vi "GetObjectExternalInterfaces.vi"(8 "Error In":errorcluster, 9 "Label":string, 10 "ThisObject":string, 11 "reference in":refnum<class "AppConfigJSON.lvclass">) -> (0 "Error Out":errorcluster, 1 "ObjectData":T1, 2 "Valid?":bool, 3 "reference out":refnum<class "AppConfigJSON.lvclass">)   [LabVIEW 2021, in "AppConfigJSON.lvclass"]
uses:
  AppConfigJSON.lvclass
  Interface_TAF_IApplicationConfiguration/IApplicationConfiguration/ObjectData.ctl
  d9591dce-848e-416d-bce7-ad181968b3a1.vi
  <vilib>/TriekselSoft/TracerLibrary/TracerLibrary/Tracer/protected/SendMessage.vi
  <vilib>/TriekselSoft/TracerLibrary/TracerLibrary/Tracer/protected/Timestamp.vi
  d9591dce-848e-416d-bce7-ad181968b3a1.vi/f75db090-0877-4668-94fb-75c2140b1617.vi
  <vilib>/TriekselSoft/TracerLibrary/TracerLibrary/Tracer/Tracer_Level-Warning.vi
  <vilib>/JDP Science/JSONtext/Variant to JSON Text.vi
  <vilib>/TriekselSoft/TracerLibrary/TracerLibrary/Tracer/protected/Tracer_ClassAttributes.vi
  <vilib>/JDP Science/JSONtext/LVClass Serializer/JSONtext LVClass Serializer.lvclass
  Interface_TAF_IApplicationConfiguration/IApplicationConfiguration/IApplicationConfiguration.lvclass
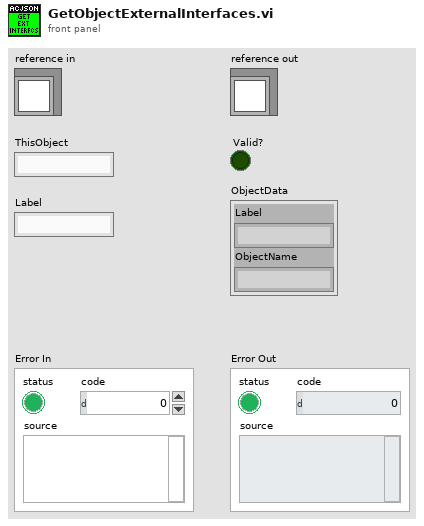
[diagram p1: front panel]
types:
  T1 = typedef "IApplicationConfiguration.lvclass/ObjectData.ctl" = cluster{"Label":string, "ObjectName":string}
  T2 = typedef "AppConfigJSON.lvclass/ObjectAttributes.ctl" = cluster{"Name":string, "ConfigFilePath":path, "Objects":T3[], "ApplicationBasePath":path}
  T3 = typedef "IApplicationConfiguration.lvclass/ObjectDataDetails.ctl" = cluster{"ObjectName":string, "ObjectType":string, "Interfaces":T1[]}
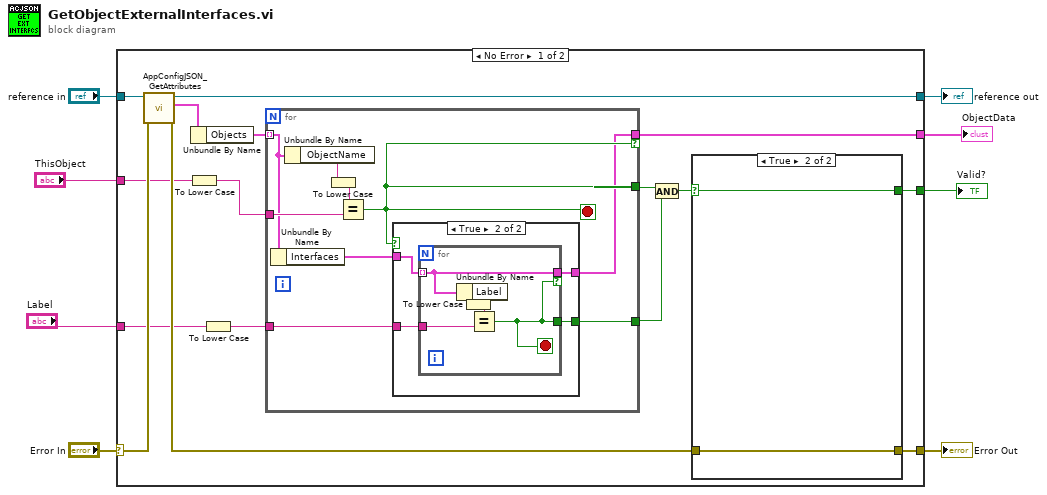
[diagram p0: block diagram]
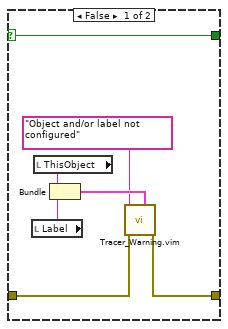
[diagram p2: hidden frame]
diagram:
  n1 = case shown="No Error" "Error In" {
    selector: "Error In" -> [w24 w53]
    tunnel: [w16 w53] -> w7
    tunnel: [w21 w52] -> w5
    tunnel: "reference in" -> [w22 w52]
    tunnel: "ThisObject" -> [w10 _]
    tunnel: [w18 _] -> w3
    tunnel: "Label" -> [w14 _]
    tunnel: [w9 _] -> w1
    frame No Error {
      n2 = call "AppConfigJSON_GetAttributes.vi"("error in (no error)"=w24, "reference in"=w22) -> ("error out"=w15:errorcluster, "Data"=w23:T2, "reference out"=w21:refnum<class "AppConfigJSON.lvclass">)  [unwired: 6 in, 1 out]
      n3 = To Lower Case(string=w10) -> (all lower case string=w19:string)
      n4 = Unbundle By Name(w23) -> ("Objects"=w20:T3[])
      n5 = To Lower Case(string=w14) -> (all lower case string=w13:string)
      n6 = for {
        tunnel: w19 -> [w42]
        tunnel: w20 -> [w38] mode=indexing
        tunnel: [w35] -> w18 if=w39
        tunnel: [w39] -> w17
        tunnel: w13 -> [w36]
        tunnel: [w34] -> w11
        stop <- w39 stop-if-true
        n7 = Unbundle By Name(w38) -> ("Interfaces"=w37:T1[])
        n8 = Unbundle By Name(w38) -> ("ObjectName"=w41:string)
        n9 = To Lower Case(string=w41) -> (all lower case string=w40:string)
        n10 = Equal?(x=w40, y=w42) -> (x = y?=w39:bool)
        n11 = case shown="True" w39 {
          tunnel: w37 -> [_ w46]
          tunnel: w36 -> [_ w45]
          tunnel: [_ w44] -> w35
          tunnel: [_ w43] -> w34
          frame False {
          }
          frame True {
            n12 = for {
              tunnel: w46 -> [w48] mode=indexing
              tunnel: w45 -> [w49]
              tunnel: [w48] -> w44 if=w47
              tunnel: [w47] -> w43
              stop <- w47 stop-if-true
              n13 = Unbundle By Name(w48) -> ("Label"=w51:string)
              n14 = To Lower Case(string=w51) -> (all lower case string=w50:string)
              n15 = Equal?(x=w50, y=w49) -> (x = y?=w47:bool)
            }
          }
        }
      }
      n16 = And(x=w17, y=w11) -> (x .and. y?=w12:bool)
      n17 = case shown="True" w12 {
        selector: w12 -> [w25 w32]
        tunnel: w15 -> [w27 w33]
        tunnel: [w26 w33] -> w16
        tunnel: [w25 w32] -> w9
        frame False {
          n18 = local read "Label"() -> (w28:string)
          n19 = local read "ThisObject"() -> (w29:string)
          n20 = Bundle("ThisObject"=w29, "Label"=w28) -> (w31:cluster{"ThisObject":string, "Label":string})  [unwired: 1 in]
          n21 = call "Tracer_Warning.vim"("Data"=w31, "error in (no error)"=w27, "WarningText"="Object and/or label not configured") -> ("error out"=w26:errorcluster)  [unwired: 8 in]
        }
        frame True {
        }
      }
    }
    frame Error {
    }
  }
  "Error Out" <- w7
  "reference out" <- w5
  "ObjectData" <- w3
  "Valid?" <- w1
